vi "_FPGA Turbo Control.vi"(6 "error in (no error)":errorcluster, 8 "Command":T1=enum."Read Actual Rotation Speed in Hz") -> (0 "error out":errorcluster, 1 "Speed":i32, 2 "Reply":string, 4 "Error Code":string, 5 "Time":i32)   [LabVIEW 2015]
uses:
  Type/_Pump Parameter.ctl
  Type/_RT Serial Command.ctl
  _RT Global.vi
  <vilib>/Utility/error.llb/Error Cluster From Error Code.vi
  <vilib>/rvi/errors/niLvFpgaAdjustHostInterfaceError.vi
  <vilib>/rvi/interface/nirviReadWriteControl/nirviReadWriteControl.xnode
  Type/FPGA Typedef.ctl
  FPGA Bitfiles/FPGA9607.lvbitx
  NiFpgaLv.dll
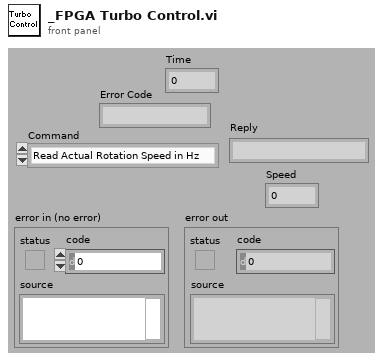
[diagram p1: front panel]
types:
  T1 = typedef "_Pump Parameter.ctl" = enum16{"Turn Pump Motor On", "Turn Pump Motor Off", "Read Pump Oil Deficiency", "Read Rotation Switch Point Attained", "Read Ele. Drive Over Temperature", "Read Pump Over Temperature", "Read Set Rotation Speed Attained", "Read Turbopump Accelerates", "Read Actual Rotation Speed in Hz", "Read Motor Current in A", "Read Operating Hours in h", "Read Motor Voltage in V", "Read Motor Power in W", "Set Rotation Speed Switchpoint in %", "Clear Error", "Read Error Code", "Read Bearing Temperature", "Read Hardware Version", "Read Firmware Version", "Read Operating Hours (Drive)", "Read Rotational Speed (rpm)", "Read Power Stage Temperature", "Read Electronics Temperature", "Read Upper Pump Temperature", "Read Motor Temperature", "Read Error Code History, 1", "Read Error Code History, 2", "Read Error Code History, 3", "Read Error Code History, 4", "Read Error Code History, 5", "Read Error Code History, 6", "Read Error Code History, 7", "Read Error Code History, 8", "Read Error Code History, 9", "Read Error Code History, 10"}
  T2 = typedef "_RT Serial Command.ctl" = cluster{"Port Type":u16, "baud rate (9600)":u32, "data bits (8)":u16, "stop bits (1)":u16, "parity (0:none)":u16, "DoRead":bool, "Command":string}
  T3 = typedef "FPGA Typedef.ctl" = refnum<k20>
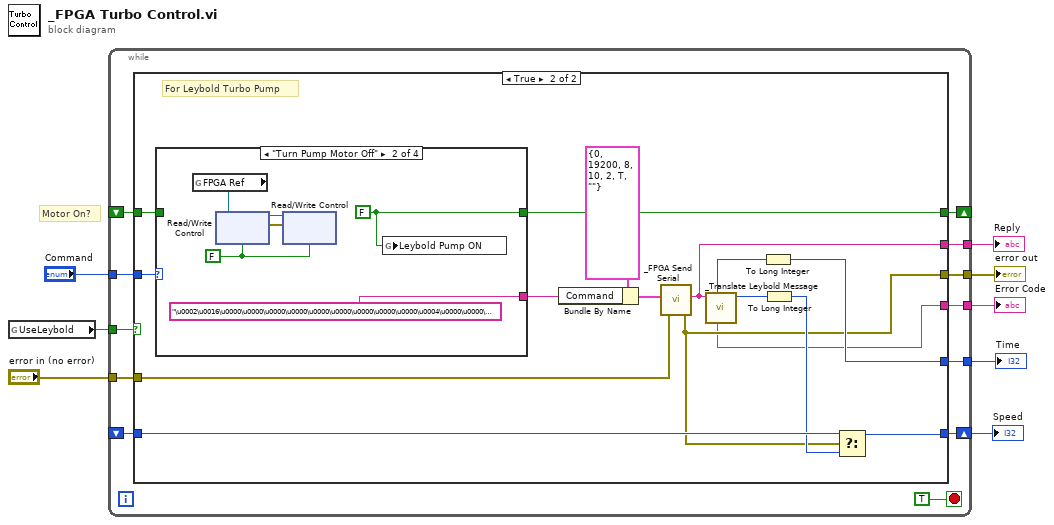
[diagram p0: block diagram]
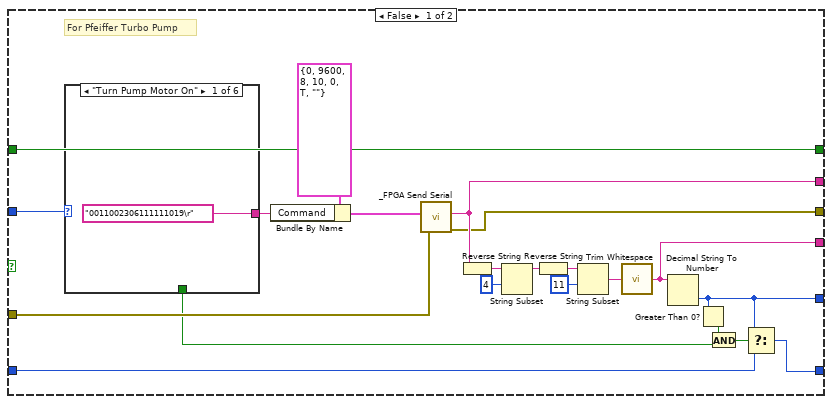
[diagram p2: hidden frame]
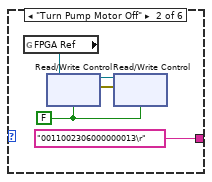
[diagram p3: hidden frame]
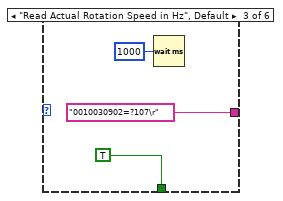
[diagram p4: hidden frame]
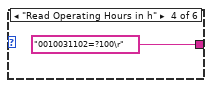
[diagram p5: hidden frame]
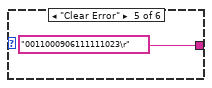
[diagram p6: hidden frame]
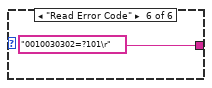
[diagram p7: hidden frame]
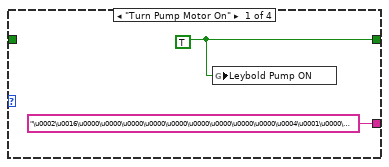
[diagram p8: hidden frame]
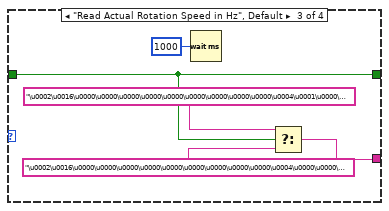
[diagram p9: hidden frame]
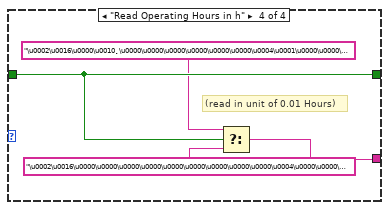
[diagram p10: hidden frame]
diagram:
  # "Motor On?"
  n1 = global read "_RT Global.vi" "UseLeybold"() -> (w3:bool)
  n2 = while {
    tunnel: [w19] -> w7
    tunnel: [w18] -> w6
    tunnel: [w17] -> w5
    tunnel: "Command" -> [w16]
    tunnel: w3 -> [w15]
    tunnel: "error in (no error)" -> [w14]
    tunnel: [w13] -> w1
    shift-right: [w20] -> w8
    shift-left: _ -> [w11]
    shift-right: [w10] -> _
    shift-left: _ -> [w9]
    stop <- TRUE stop-if-true
    n3 = case shown="True" w15 {
      tunnel: [w41 w58] -> w20
      tunnel: [w40 w61] -> w19
      tunnel: [w39 w54] -> w18
      tunnel: [w38 w55] -> w17
      tunnel: w16 -> [w37 w69]
      tunnel: w14 -> [w36 w56]
      tunnel: [w35 w57] -> w13
      tunnel: w11 -> [w34 w60]
      tunnel: [w21 w65] -> w10
      tunnel: w9 -> [w21 w64]
      frame False {
        # "For Pfeiffer Turbo Pump"
        n4 = case shown="\"Turn Pump Motor On\"" w37 {
          tunnel: ["0011002306111111019\r" ("Command") "0011002306000000013\r" ("Command") "0010030902=?107\r" ("Command") "0010031102=?100\r" ("Command") "0011000906111111023\r" ("Command") "0010030302=?101\r" ("Command")] -> w32
          tunnel: [_ _ TRUE _ _ _] -> w24
          frame "Turn Pump Motor On" {
          }
          frame "Turn Pump Motor Off" {
            w46 = FALSE
            n5 = global read "_RT Global.vi" "FPGA Ref"() -> (w43:T3)
            n6 = xnode "Read/Write Control"("FPGA VI Reference In"=w43, "FilaB"=w46) -> ("FPGA VI Reference Out"=w44:T3, "error out"=w45:errorcluster)  [unwired: 1 in]
            n7 = xnode "Read/Write Control"("FPGA VI Reference In"=w44, "error in"=w45, "FilaC"=w46) -> ()  [unwired: 2 out]
          }
          frame "Read Actual Rotation Speed in Hz", Default {
            n8 = Wait (ms)(milliseconds to wait=u32 1000) -> ()  [unwired: 1 out]
          }
          frame "Read Operating Hours in h" {
          }
          frame "Clear Error" {
          }
          frame "Read Error Code" {
          }
        }
        n9 = Bundle By Name(cluster=T2 {"Port Type"=0, "baud rate (9600)"=9600, "data bits (8)"=8, "stop bits (1)"=10, "parity (0:none)"=0, "DoRead"=TRUE, "Command"=""}, "Command"=w32) -> (w31:T2)
        n10 = call "_FPGA Send Serial.vi"("error in"=w36, "Serial Command"=w31) -> ("error out"=w35:errorcluster, "Reply"=w38:string)  [unwired: 2 in, 2 out]
        n11 = Reverse String(1:w38) -> (0:w22:string)
        n12 = String Subset(string=w22, offset (0)=4) -> (substring=w27:string)  [unwired: 1 out]
        n13 = Reverse String(1:w27) -> (0:w28:string)
        n14 = String Subset(string=w28, offset (0)=11) -> (substring=w26:string)  [unwired: 1 out]
        n15 = call <vilib>:"Trim Whitespace.vi"("string"=w26) -> ("trimmed string"=w39:string)  [unwired: 1 in]
        n16 = Decimal String To Number(string=w39) -> (number=w40:i32)  [unwired: 3 out]
        n17 = Greater Than 0?(x=w40) -> (x > 0?=w25:bool)
        n18 = And(x=w25, y=w24) -> (x .and. y?=w23:bool)
        n19 = Select(t=w40, s=w23, f=w34) -> (s? t:f=w41:i32)
      }
      frame True {
        # "For Leybold Turbo Pump"
        n20 = case shown="\"Turn Pump Motor Off\"" w69 {
          tunnel: ["\u0002\u0016\u0000\u0000\u0000\u0000\u0000\u0000\u0000\u0000\u0000\u0004\u0001\u0000\u0000\u0000\u0000\u0000\u0000\u0000\u0000\u0000\u0000\u0011" ("Command") "\u0002\u0016\u0000\u0000\u0000\u0000\u0000\u0000\u0000\u0000\u0000\u0004\u0000\u0000\u0000\u0000\u0000\u0000\u0000\u0000\u0000\u0000\u0000\u0010" ("Command") w79 w84] -> w66
          tunnel: [w70 w72 w81 w86] -> w65
          tunnel: w64 -> [_ _ w81 w86]
          frame "Turn Pump Motor On" {
            w70 = TRUE
            n21 = global write "_RT Global.vi" "Leybold Pump ON"(w70) -> ()
          }
          frame "Turn Pump Motor Off" {
            w72 = FALSE
            w77 = FALSE
            n22 = global read "_RT Global.vi" "FPGA Ref"() -> (w74:T3)
            n23 = xnode "Read/Write Control"("FPGA VI Reference In"=w74, "FilaB"=w77) -> ("FPGA VI Reference Out"=w75:T3, "error out"=w76:errorcluster)  [unwired: 1 in]
            n24 = xnode "Read/Write Control"("FPGA VI Reference In"=w75, "error in"=w76, "FilaC"=w77) -> ()  [unwired: 2 out]
            n25 = global write "_RT Global.vi" "Leybold Pump ON"(w72) -> ()
          }
          frame "Read Actual Rotation Speed in Hz", Default {
            n26 = Wait (ms)(milliseconds to wait=u32 1000) -> ()  [unwired: 1 out]
            n27 = Select(t="\u0002\u0016\u0000\u0000\u0000\u0000\u0000\u0000\u0000\u0000\u0000\u0004\u0001\u0000\u0000\u0000\u0000\u0000\u0000\u0000\u0000\u0000\u0000\u0011" ("Command"), s=w81, f="\u0002\u0016\u0000\u0000\u0000\u0000\u0000\u0000\u0000\u0000\u0000\u0004\u0000\u0000\u0000\u0000\u0000\u0000\u0000\u0000\u0000\u0000\u0000\u0010" ("Command")) -> (s? t:f=w79:string)
          }
          frame "Read Operating Hours in h" {
            # "(read in unit of 0.01 Hours)"
            n28 = Select(t="\u0002\u0016\u0000\u0010¸\u0000\u0000\u0000\u0000\u0000\u0000\u0004\u0001\u0000\u0000\u0000\u0000\u0000\u0000\u0000\u0000\u0000\u0000¹" ("Command"), s=w86, f="\u0002\u0016\u0000\u0000\u0000\u0000\u0000\u0000\u0000\u0000\u0000\u0004\u0000\u0000\u0000\u0000\u0000\u0000\u0000\u0000\u0000\u0000\u0000\u0010" ("Command")) -> (s? t:f=w84:string)
          }
        }
        n29 = Bundle By Name(cluster=T2 {"Port Type"=0, "baud rate (9600)"=19200, "data bits (8)"=8, "stop bits (1)"=10, "parity (0:none)"=2, "DoRead"=TRUE, "Command"=""}, "Command"=w66) -> (w67:T2)
        n30 = call "_FPGA Send Serial.vi"("error in"=w56, "Serial Command"=w67) -> ("error out"=w57:errorcluster, "Reply"=w55:string)  [unwired: 2 in, 2 out]
        n31 = call "_Translate Leybold Message.vi"("LeyboldMessage"=w55) -> ("Frequency"=w63:u16, "Error"=w54:string, "Parameter"=w62:u32)  [unwired: 3 in, 5 out]
        n32 = To Long Integer(number=w62) -> (32bit integer=w61:i32)
        n33 = To Long Integer(number=w63) -> (32bit integer=w59:i32)
        n34 = Select(t=w60, s=w57, f=w59) -> (s? t:f=w58:i32)
      }
    }
  }
  "Speed" <- w8
  "Time" <- w7
  "Error Code" <- w6
  "Reply" <- w5
  "error out" <- w1
